vi "SLAM_Testing.vi"() -> ()   [LabVIEW 2012]
uses:
  <vilib>/DAQmx/write.llb/DAQmx Write.vi
  <vilib>/DAQmx/write.llb/DAQmx Write (Digital 1D Bool NChan 1Samp 1Line).vi
  <vilib>/DAQmx/configure/task.llb/DAQmx Clear Task.vi
  <vilib>/DAQmx/create/task.llb/DAQmx Create Task.vi
  <vilib>/DAQmx/configure/task.llb/DAQmx Start Task.vi
  <vilib>/DAQmx/create/channels.llb/DAQmx Create Virtual Channel.vi
  <vilib>/DAQmx/create/channels.llb/DAQmx Create Channel (DO-Digital Output).vi
  <vilib>/DAQmx/miscellaneous.llb/DAQmx Fill In Error Info.vi
panel:
  in  "File Name":string
  in  "Save Enable":bool
  in  "Timed Relay Control":bool
  in  "ECOLAB Button":bool
  in  "Tab Control":enum32{"MAIN", "  CONFIG  "}(tab)
  out "Flow2 Wayne":dbl
  out "Vol Percent":dbl format="%.1f"
  in  "Save When Running?":bool=TRUE
  out "Ave FLOW Ratio":dbl format="%.1f"
  out "Ave VDC2":dbl format="%.1f"
  out "Ave VDC1":dbl format="%.1f"
  out "VOLTAGE 2":dbl format="%.1f"
  out "FLOW 2":u32
  in  "ENABLE OUTPUT":bool
  in  "Time Setpoint [s]":dbl=10.0
  in  "START/RESET":bool
  out "MASS 1":dbl format="%.1f"
  out "MASS 2":dbl format="%.1f"
  out "VOLTAGE 1":dbl format="%.1f"
  out "Elapsed Time [s]":dbl format="%.1f"
  out "Output":bool
  out "FLOW 1":u32
  in  "Reset Flow 1":bool
  in  "Reset Flow 2":bool
  in  "Average Interval [sec]":dbl=0.1
  in  "X Seconds":dbl=3.0
  out "Ave Size":i32=86
  out "Flow1 Wayne":dbl
  in  "DAQ TAB":T1(tab)=enum."9237"
  in  "Save Interval [s]":dbl=1.0 min=0.0
  in  "Folder Location":path
  out "Save Error":errorcluster
  out "File Path":path
  in  "Scale Template":T2={"Channel Select"=0, "Clear/Reset Scales"=FALSE, "Channel #"=["0", "1", "2", "3", "4", "5"], "Scale Names"=["0", "1", "2", "3", "4", "5"], "Set?"=[FALSE, FALSE, FALSE, FALSE, FALSE, FALSE, FALSE, FALSE, FALSE, FALSE, FALSE, FALSE], "HI/LO Setpoints"=[1.0, 0.0, 1.0, 0.0, 1.0, 0.0, 1.0, 0.0, 1.0, 0.0, 1.0, 0.0], "Units"=["0", "1", "2", "3", "4", "5"], "HI/LO Signals"=[1.0, 0.0, 1.0, 0.0, 1.0, 0.0, 1.0, 0.0, 1.0, 0.0, 1.0, 0.0], "Slope/Intercept"=[1.0, 0.0, 1.0, 0.0, 1.0, 0.0, 1.0, 0.0, 1.0, 0.0, 1.0, 0.0], "IN/OUT Values"=[0.0, 0.0, 0.0, 0.0, 0.0, 0.0, 0.0, 0.0, 0.0, 0.0, 0.0, 0.0], "Sim Signals?"=FALSE, "Sim. Signal"=0.0} {"Sim. Signal" format="%#.3p"; "Channel Select" min=0 step=1; "Slope/Intercept" format="%#.3p"; "HI/LO Setpoints" format="%#.3p"; "IN/OUT Values" format="%#.3p"; "HI/LO Signals" format="%#.3p"}
  in  "9237 Name":tag="9237"
  in  "9237 Config":T3={"Sample Rate [Hz]"=25000.0, "Number of Samples"=2500, "Max Value [V]"=0.025, "Min Value [V]"=-0.025, "Voltage Excitation Source"=10200, "Ext. Excitation Value (VDC)"=10.0, "Sample Timing Index"=0, "Cut-Off [Hz]"=1.0, "HI/LO Trim [%]"=10.0, "Near Stable Threshold [V]"=1e-06, "Near Stable Change Limit [V]"=5e-07, "Stable Threshold [V]"=2.5e-08, "Stable Change Limit [V]"=1e-10, "Rolling Average"=4} {"Voltage Excitation Source" items=["Internal"=10200, "External"=10167, "None"=10230]; "Sample Timing Index" max=2; "Sample Rate [Hz]" format="%#_6p"; "Max Value [V]" format="%#_6p"; "Min Value [V]" format="%#_6p"; "Stable Change Limit [V]" format="%.2p"; "Stable Threshold [V]" format="%.2p"; "Near Stable Change Limit [V]" format="%.2p"; "Near Stable Threshold [V]" format="%.2p"; "Cut-Off [Hz]" format="%0.2f"}
  out "9237 Error":errorcluster={"status"=TRUE, "code"=-200077, "source"="Property Node DAQmx Timing (arg 1) in DAQmx 9237 4ch Load Cell (SubVI).vi->SLAM_Testing.vi <append>\n<B>Property: </B>SampTimingEngine\n<B>Requested Value: </B>0\n<B>You Can Select: </B>2\n\n<B>Task Name: </B>9237"}
  in  "9229 Name":tag="9229"
  in  "9229 Config":T4={"Sample Rate [Hz]"=25000.0, "Samples/Ch"=2500, "Max Value [V]"=60.0, "Min Value [V]"=0.0, "Rolling Average"=5, "HI/LO Trim [%]"=1.0, "Sample Timing Engine"=2} {"Sample Timing Engine" max=2; "Sample Rate [Hz]" min=0.0001 max=50000.0 format="%#_6p"; "Samples/Ch" min=1 step=1; "Max Value [V]" min=-60.0 max=60.0 format="%#_6p"; "Min Value [V]" min=-60.0 max=60.0 format="%#_6p"; "Rolling Average" min=1 step=1; "HI/LO Trim [%]" min=1.0 max=99.0}
  out "9229 Error":errorcluster={"status"=TRUE, "code"=-200220, "source"="SLAM_Testing.vi<append>\n<B>Device Specified: </B>9229\n<B>Suggested Device(s): </B>cDAQ5, 9237, 6009\n\n<B>Task Name: </B>9229"}
  in  "9411 Name":tag="9411"
  out "9411 Error":errorcluster={"status"=TRUE, "code"=-201003, "source"="DAQmx Create Channel (CI-Count Edges).vi:2<append>\n<B>Device Specified: </B>9411\n\n<B>Task Name: </B>9411_0"}
  in  "K-Factor Array [pulses / liter]":dbl[](array[numeric])=[1800.0, 1800.0, 1800.0, 1800.0]
  in  "Reset Array":bool[](array[boolean])=[FALSE, FALSE, FALSE, FALSE]
  out "Flow0":T5 {"Volume [gal]" format="%#.3f"; "Rate [GPM]" format="%#.3f"; "Elapsed Time [s]" format="%.1f"}
  out "Flow1":T5 {"Volume [gal]" format="%#.3f"; "Rate [GPM]" format="%#.3f"; "Elapsed Time [s]" format="%.1f"}
  out "Flow2":T5 {"Volume [gal]" format="%#.3f"; "Rate [GPM]" format="%#.3f"; "Elapsed Time [s]" format="%.1f"}
  in  "9411 Config":T6={"Digital Filter Enable"=TRUE, "Minimum Pulse Width [seconds]"=2.5e-08} {"Minimum Pulse Width [seconds]" min=2.5e-08 max=6.4e-06 format="%.3p"}
  out "Flow3":T5 {"Volume [gal]" format="%#.3f"; "Rate [GPM]" format="%#.3f"; "Elapsed Time [s]" format="%.1f"}
  in  "Relay Control (Manual)":bool[](array[boolean])=[FALSE, FALSE, FALSE, FALSE]
  out "9481 Error":errorcluster
  in  "9481 Name":tag="9481"
  in  "Stop Program":bool=TRUE
  # "Hand Care Concentrates"
  # "Save Enable"
  # "File / Test Name"
  # "Blake Otting 6-26-2013"
  # "TEST CONTROL"
  # "TEST MEASUREMENTS"
  # "LIVE MEASUREMENTS"
  # "grams"
  # "Average Values"
  # "grams"
  # "Voltage 1"
  # "vdc"
  # "Voltage 2"
  # "vdc"
  # "vdc"
  # "Volume Ratio"
  # "vdc"
  # "Flow1 / Flow2"
  # "Volume %"
  # "Flow2 / (F1+F2)"
  # "mL"
  # "Scaled Output Value"
  # "mL"
  # "Stop Saving\nN seconds after OFF"
  # "Save When Enabled\nand Running + N?"
  # "Scaled Output Value"
  # "0 = Use Manual Save Signal Only"
  # "Ch.\n#"
  # "Scale\nName"
  # "Set\nValues?"
  # "Channel\nSelect"
  # "Scaled"
  # "Pre-Scaled"
  # "Scaling Result"
  # "Values"
  # "Units"
  # "Values"
  # "HI"
  # "Slope"
  # "IN"
  # "LO"
  # "Intercept"
  # "OUT"
  # "HI"
  # "Slope"
  # "IN"
  # "LO"
  # "Intercept"
  # "OUT"
  # "HI"
  # "Slope"
  # "IN"
  # "LO"
  # "Intercept"
  # "OUT"
  # "HI"
  # "Slope"
  # "IN"
  # "LO"
  # "Intercept"
  # "OUT"
  # "DATA SAMPLE CONFIG"
  # "FILTER / SMOOTHING CONFIG"
  # "9229 Configuration"
  # "CTR0:  SRC(1)  GATE(2)  COM(12)"
  # "CTR1:  SRC(6)  GATE(7)  COM(12)"
  # "CTR2:  SRC(3)  GATE(1)  COM(12)"
  # "CTR3:  SRC(8)  GATE(6)  COM(12)"
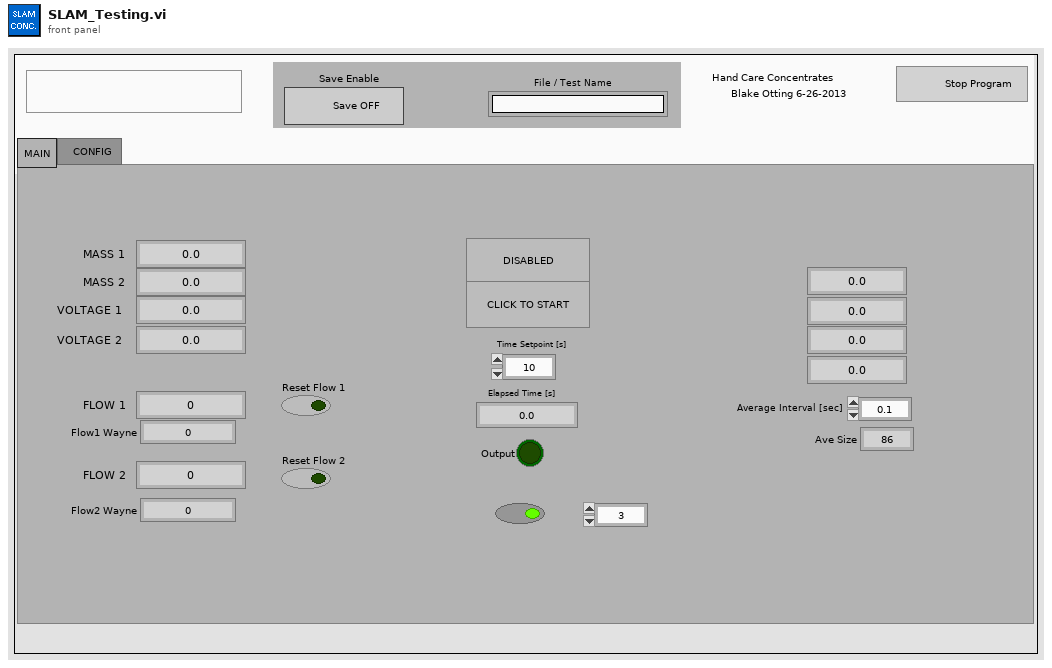
[diagram p1: front panel]
types:
  T1 = enum32{"SAVE", "SCALE", "9237", "9229", "9411", "9481"}
  T2 = cluster{"Channel Select":i32, "Clear/Reset Scales":bool, "Channel #":string[], "Scale Names":string[], "Set?":bool[], "HI/LO Setpoints":dbl[], "Units":string[], "HI/LO Signals":dbl[], "Slope/Intercept":dbl[], "IN/OUT Values":dbl[], "Sim Signals?":bool, "Sim. Signal":dbl}
  T3 = cluster{"Sample Rate [Hz]":dbl, "Number of Samples":i32, "Max Value [V]":dbl, "Min Value [V]":dbl, "Voltage Excitation Source":i32, "Ext. Excitation Value (VDC)":dbl, "Sample Timing Index":u32, "Cut-Off [Hz]":dbl, "HI/LO Trim [%]":dbl, "Near Stable Threshold [V]":dbl, "Near Stable Change Limit [V]":dbl, "Stable Threshold [V]":dbl, "Stable Change Limit [V]":dbl, "Rolling Average":i32}
  T4 = cluster{"Sample Rate [Hz]":dbl, "Samples/Ch":i32, "Max Value [V]":dbl, "Min Value [V]":dbl, "Rolling Average":i32, "HI/LO Trim [%]":dbl, "Sample Timing Engine":u32}
  T5 = cluster{"Pulse Count":u32, "Volume [mL]":u32, "Volume [gal]":dbl, "Rate [GPM]":dbl, "Elapsed Time [s]":dbl}
  T6 = cluster{"Digital Filter Enable":bool, "Minimum Pulse Width [seconds]":dbl}
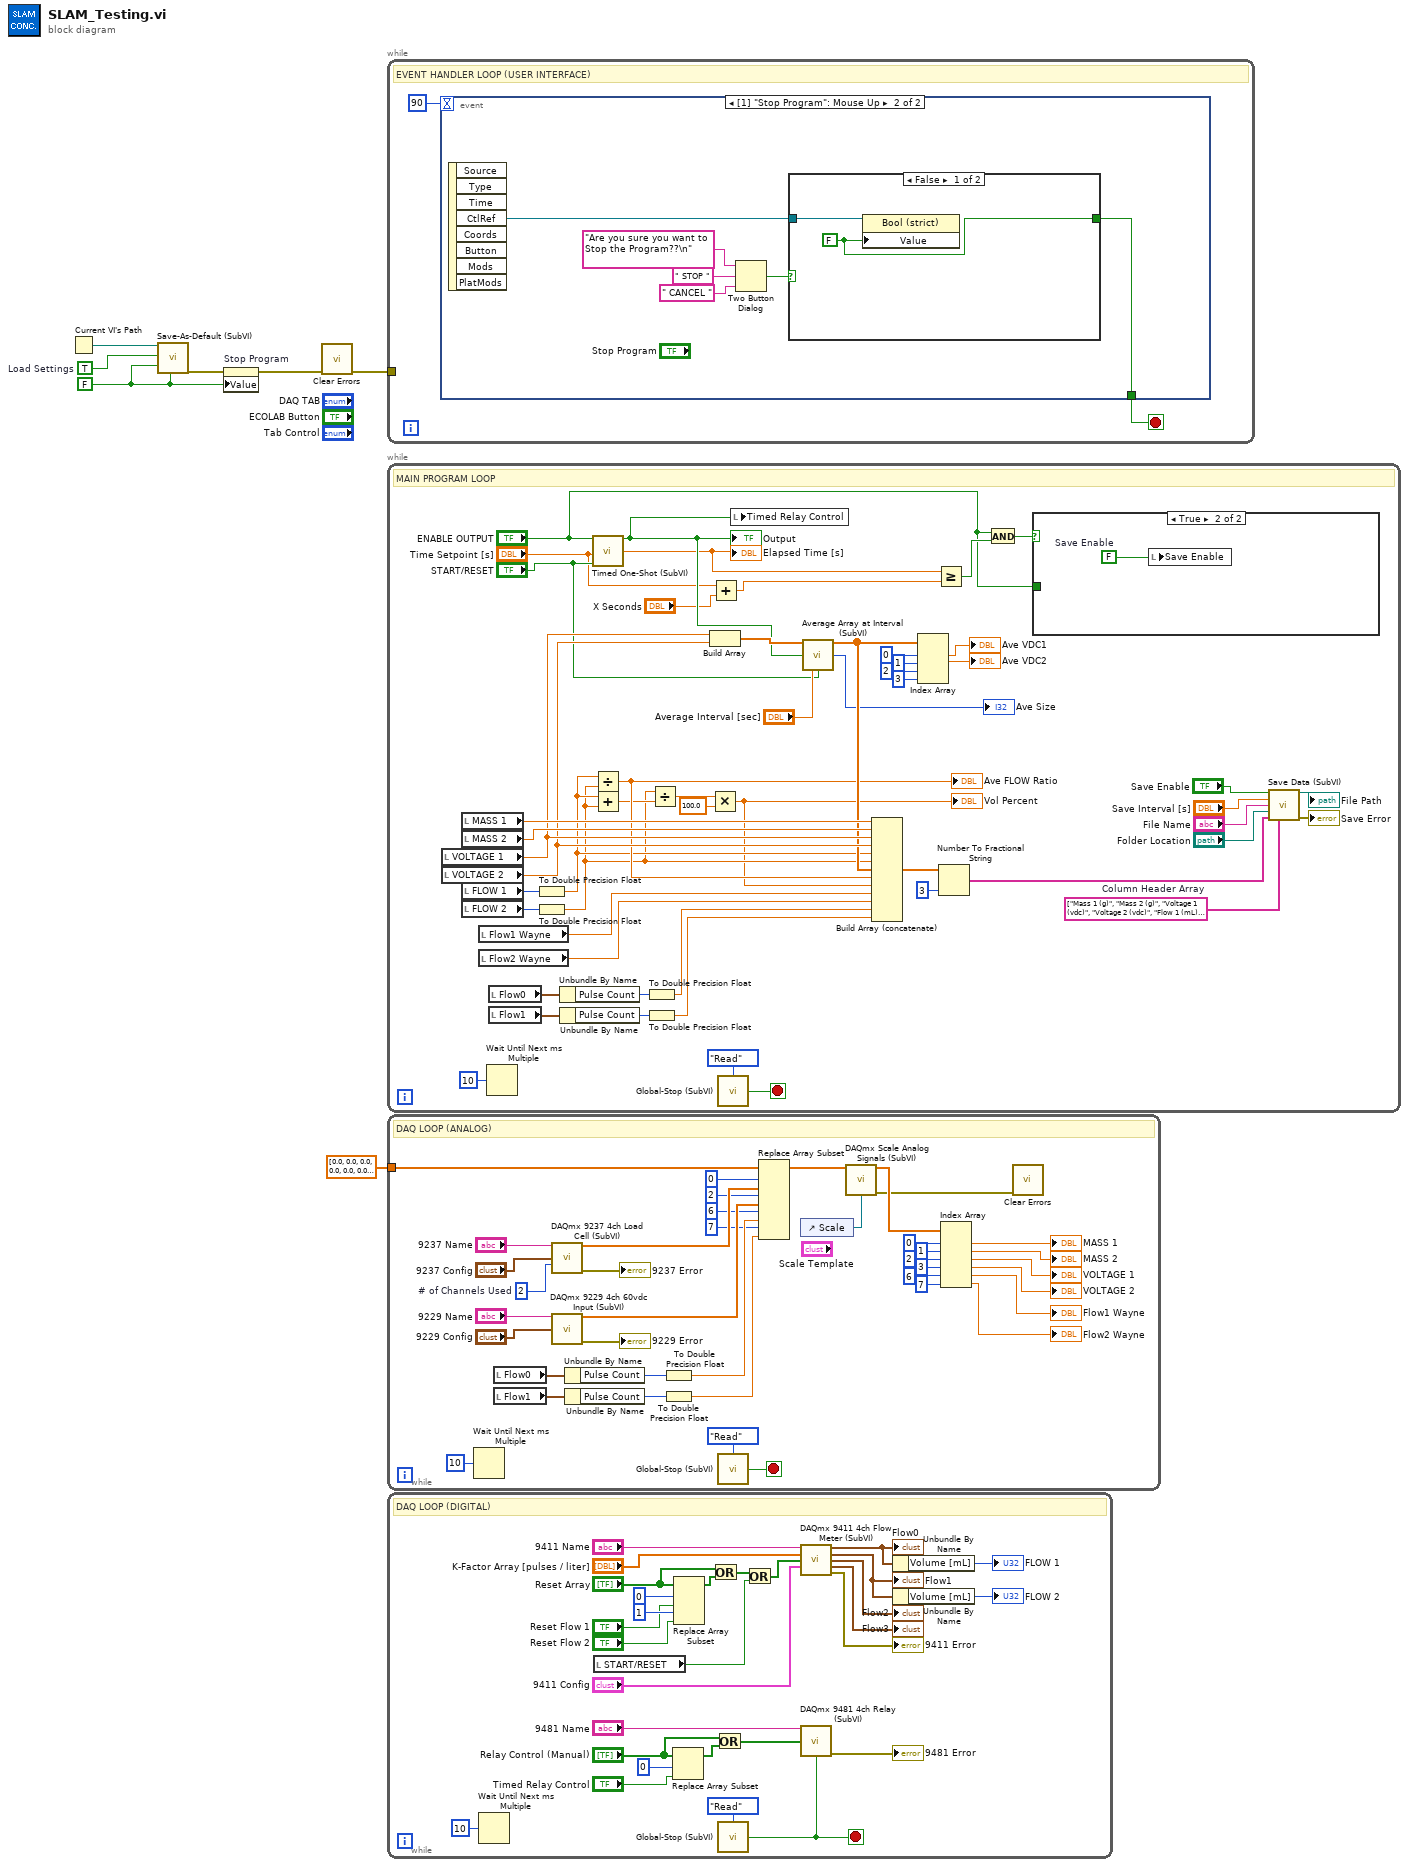
[diagram p0: block diagram]
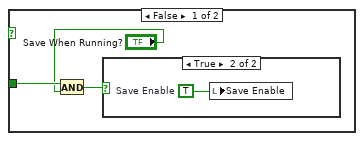
[diagram p2: hidden frame]
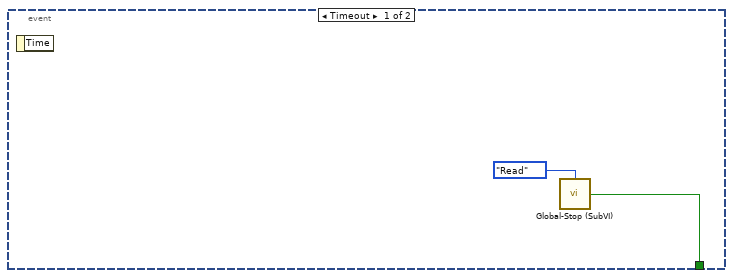
[diagram p4: hidden frame]
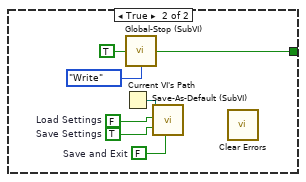
[diagram p5: hidden frame]
diagram:
  w4 = TRUE  # Load Settings
  w2 = FALSE
  n1 = Current VI's Path() -> (path=w5:path)
  n2 = call "Save-As-Default (SubVI).vi"("Current VI's Path"=w5, "Load Settings"=w4, "Save Settings"=w2, "Save and Exit"=w2) -> ("Save as Default Error"=w3:errorcluster)  [unwired: 15 in]
  n3 = property on="Stop Program" class="Bool (strict)"(error in=w3, "Value"=w2) -> (error out=w7:errorcluster)  [unwired: 1 in, 1 out]
  n4 = call <vilib>:"Clear Errors.vi"("error in (no error)"=w7) -> ("error out"=w6:errorcluster)  [unwired: 6 out]
  n5 = while {
    tunnel: w6 -> [_]
    stop <- w9 stop-if-true
    # "EVENT HANDLER LOOP (USER INTERFACE)"
    n6 = event shown="[1] \"Stop Program\": Mouse Up" {
      selector: _ -> [_ _]
      dyn-events: _ -> [_ _]
      timeout: 90 -> [_ _]
      tunnel: [w10 w13] -> w9
      event Timeout {
        n7 = event-data() -> ()  [unwired: 2 out]
        n8 = call "Global-Stop (SubVI).vi"("Mode (Read)"=enum16{"Read", "Write"}."Read") -> ("OUT"=w10:bool)  [unwired: 3 in]
      }
      event "Stop Program": Mouse Up {
        n9 = event-data() -> ("CtlRef"=w12:refnum<vi>)  [unwired: 8 out]
        n10 = Two Button Dialog(message="Are you sure you want to Stop the Program??\n", 1:" CANCEL " ("F button name (\"Cancel\")"), 2:" STOP ") -> (T button?=w14:bool)
        n11 = case shown="False" w14 {
          tunnel: [w18 w24] -> w13
          tunnel: w12 -> [w19 _]
          frame False {
            w18 = FALSE ("Value")
            n12 = property class="Bool (strict)"(reference=w19, "Value"=w18) -> ()  [unwired: 1 in, 2 out]
          }
          frame True {
            w20 = FALSE  # Save and Exit
            w21 = TRUE  # Save Settings
            w22 = FALSE  # Load Settings
            n13 = Current VI's Path() -> (path=w23:path)
            n14 = call "Global-Stop (SubVI).vi"("Mode (Read)"=enum16{"Read", "Write"}."Write", "IN"=TRUE) -> ("OUT"=w24:bool)  [unwired: 2 in]
            n15 = call "Save-As-Default (SubVI).vi"("Current VI's Path"=w23, "Load Settings"=w22, "Save Settings"=w21, "Save and Exit"=w20) -> ()  [unwired: 15 in, 1 out]
            n16 = call <vilib>:"Clear Errors.vi"() -> ()  [unwired: 1 in, 7 out]
          }
        }
      }
    }
  }
  n17 = while {
    stop <- w78 stop-if-true
    w68 = string[] ["Mass 1 (g)", "Mass 2 (g)", "Voltage 1 (vdc)", "Voltage 2 (vdc)", "Flow 1 (mL)", "Flow 2 (mL)", "Ave VDC1", "Ave VDC2", "Ave Flow Ratio", "Ave Percentage", "Flow1 Wayne", "Flow2 Wayne", "Flow0 Raw Pulse", "Flow1 Raw Pulse"]  # Column Header Array
    # "MAIN PROGRAM LOOP"
    n18 = local read "VOLTAGE 1"() -> (w62:dbl)
    n19 = local read "VOLTAGE 2"() -> (w61:dbl)
    n20 = local read "MASS 1"() -> (w76:dbl)
    n21 = local read "MASS 2"() -> (w75:dbl)
    n22 = local read "FLOW 1"() -> (w74:u32)
    n23 = local read "FLOW 2"() -> (w73:u32)
    n24 = local read "Flow1 Wayne"() -> (w32:dbl)
    n25 = local read "Flow2 Wayne"() -> (w31:dbl)
    n26 = Wait Until Next ms Multiple(millisecond multiple=u32 10) -> ()  [unwired: 1 out]
    n27 = local read "Flow0"() -> (w33:T5)
    n28 = local read "Flow1"() -> (w34:T5)
    n29 = To Double Precision Float(number=w74) -> (double precision float=w40:dbl)
    n30 = To Double Precision Float(number=w73) -> (double precision float=w38:dbl)
    n31 = Unbundle By Name(w33) -> ("Pulse Count"=w30:u32)
    n32 = Unbundle By Name(w34) -> ("Pulse Count"=w29:u32)
    n33 = call "Timed One-Shot (SubVI).vi"("ENABLE OUTPUT"="ENABLE OUTPUT", "Time Setpoint [s]"="Time Setpoint [s]", "START/RESET"="START/RESET") -> ("Output"=w50:bool, "Elapsed Time [s]"=w49:dbl)  [unwired: 11 in]
    "Elapsed Time [s]" <- w49
    "Output" <- w50
    n34 = Divide(x=w40, y=w38) -> (x/y=w41:dbl)
    "Ave FLOW Ratio" <- w41
    n35 = Add(x=w40, y=w38) -> (x+y=w39:dbl)
    n36 = To Double Precision Float(number=w30) -> (double precision float=w28:dbl)
    n37 = To Double Precision Float(number=w29) -> (double precision float=w27:dbl)
    n38 = Divide(x=w38, y=w39) -> (x/y=w37:dbl)
    n39 = Build Array(w62, w61) -> (w60:dbl[])
    n40 = Multiply(x=w37, y=100.0) -> (x*y=w35:dbl)
    "Vol Percent" <- w35
    n41 = Add(x="Time Setpoint [s]", y="X Seconds") -> (x+y=w45:dbl)
    n42 = call "Global-Stop (SubVI).vi"("Mode (Read)"=enum16{"Read", "Write"}."Read") -> ("OUT"=w78:bool)  [unwired: 3 in]
    n43 = local write "Timed Relay Control"(w50) -> ()
    n44 = call "Average Array at Interval (SubVI).vi"("Signals IN"=w60, "Enable"=w50, "Sample Interval [sec]"="Average Interval [sec]", "Reset Averages"="START/RESET") -> ("Signals OUT"=w53:dbl[], "Ave Size"=→"Ave Size":i32)  [unwired: 10 in]
    n45 = Build Array (concatenate)(w76, w75, w62, w61, w40, w38, w53, w41, w35, w32, w31, w28, w27) -> (w64:dbl[])
    n46 = Index Array(array=w53, index #1=0, index #2=1, index #3=2, index #4=3) -> (element #1=→"Ave VDC1":dbl, element #2=→"Ave VDC2":dbl)  [unwired: 2 out]
    n47 = Greater Or Equal?(x=w49, y=w45) -> (x >= y?=w44:bool)
    n48 = Number To Fractional String(number=w64, precision (6)=i16 3) -> (F-format string=w70:string[])  [unwired: 2 in]
    n49 = And(x="ENABLE OUTPUT", y=w44) -> (x .and. y?=w43:bool)
    n50 = case shown="True" w43 {
      tunnel: "ENABLE OUTPUT" -> [w82 _]
      frame False {
        n51 = And(x=w82, y="Save When Running?") -> (x .and. y?=w80:bool)
        n52 = case shown="True" w80 {
          frame False {
          }
          frame True {
            w83 = TRUE  # Save Enable
            n53 = local write "Save Enable"(w83) -> ()
          }
        }
      }
      frame True {
        w84 = FALSE  # Save Enable
        n54 = local write "Save Enable"(w84) -> ()
      }
    }
    n55 = call "Save Data (SubVI).vi"("Save Enable"="Save Enable", "Save Interval [sec]"="Save Interval [s]", "File Name"="File Name", "Folder Location"="Folder Location", "Data Array (Row)"=w70, "Column Header Array"=w68) -> ("File Path"=→"File Path":path, "Save Error"=→"Save Error":errorcluster)  [unwired: 7 in, 1 out]
  }
  n56 = while {
    tunnel: dbl[] [0.0, 0.0, 0.0, 0.0, 0.0, 0.0, 0.0, 0.0] -> [w113]
    stop <- w122 stop-if-true
    w99 = 2  # # of Channels Used
    # "DAQ LOOP (ANALOG)"
    n57 = Wait Until Next ms Multiple(millisecond multiple=u32 10) -> ()  [unwired: 1 out]
    n58 = local read "Flow0"() -> (w86:T5)
    n59 = local read "Flow1"() -> (w85:T5)
    n60 = call "DAQmx 9237 4ch Load Cell (SubVI).vi"("9237 Name"="9237 Name", "9237 Config"="9237 Config", "# of Channels Used"=w99) -> ("Filtered Signals"=w121:dbl[], "9237 Error"=→"9237 Error":errorcluster)  [unwired: 8 in, 3 out]
    n61 = call "DAQmx 9229 4ch 60vdc Input (SubVI).vi"("9229 Name"="9229 Name", "9229 Config"="9229 Config") -> ("Measurements"=w117:dbl[], "9229 Error"=→"9229 Error":errorcluster)  [unwired: 12 in]
    n62 = Unbundle By Name(w86) -> ("Pulse Count"=w95:u32)
    n63 = Unbundle By Name(w85) -> ("Pulse Count"=w93:u32)
    n64 = To Double Precision Float(number=w95) -> (double precision float=w94:dbl)
    n65 = To Double Precision Float(number=w93) -> (double precision float=w91:dbl)
    n66 = call "Global-Stop (SubVI).vi"("Mode (Read)"=enum16{"Read", "Write"}."Read") -> ("OUT"=w122:bool)  [unwired: 3 in]
    n67 = Replace Array Subset(array=w113, new element #1=w121, index #1=0, new element #2=w117, index #2=2, new element #3=w94, index #3=6, new element #4=w91, index #4=7) -> (w111:dbl[])
    n68 = control-ref of="Scale"() -> (w112:refnum<vi>)
    n69 = call "DAQmx Scale Analog Signals (SubVI).vi"("Measured Signals"=w111, "Scale Reference"=w112) -> ("Scaled Values"=w110:dbl[], "Scale Error"=w100:errorcluster)  [unwired: 12 in]
    n70 = Index Array(array=w110, index #1=0, index #2=1, index #3=2, index #4=3, index #5=6, index #6=7) -> (element #1=→"MASS 1":dbl, element #2=→"MASS 2":dbl, element #3=→"VOLTAGE 1":dbl, element #4=→"VOLTAGE 2":dbl, element #5=→"Flow1 Wayne":dbl, element #6=→"Flow2 Wayne":dbl)
    n71 = call <vilib>:"Clear Errors.vi"("error in (no error)"=w100) -> ()  [unwired: 6 in, 1 out]
  }
  n72 = while {
    stop <- w150 stop-if-true
    # "DAQ LOOP (DIGITAL)"
    n73 = Wait Until Next ms Multiple(millisecond multiple=u32 10) -> ()  [unwired: 1 out]
    n74 = local read "START/RESET"() -> (w125:bool)
    n75 = Replace Array Subset(array="Relay Control (Manual)", new element="Timed Relay Control", index=0) -> (w130:bool[])
    n76 = Replace Array Subset(array="Reset Array", new element #1="Reset Flow 1", index #1=0, new element #2="Reset Flow 2", index #2=1) -> (w136:bool[])
    n77 = Or(x="Reset Array", y=w136) -> (x .or. y?=w126:bool[])
    n78 = Or(x="Relay Control (Manual)", y=w130) -> (x .or. y?=w132:bool[])
    n79 = call "Global-Stop (SubVI).vi"("Mode (Read)"=enum16{"Read", "Write"}."Read") -> ("OUT"=w150:bool)  [unwired: 3 in]
    n80 = Or(x=w126, y=w125) -> (x .or. y?=w124:bool[])
    n81 = call "DAQmx 9411 4ch Flow Meter (SubVI).vi"("9411 Name"="9411 Name", "K-Factor Array [pulses / liter]"="K-Factor Array [pulses / liter]", "Reset Array"=w124, "9411 Config"="9411 Config") -> ("Flow0"=w141:T5, "Flow1"=w142:T5, "Flow2"=→"Flow2":T5, "Flow3"=→"Flow3":T5, "9411 Error"=→"9411 Error":errorcluster)  [unwired: 7 in]
    "Flow0" <- w141
    "Flow1" <- w142
    n82 = call "DAQmx 9481 4ch Relay (SubVI).vi"("9481 Name"="9481 Name", "Relay Control"=w132, "Stop Program"=w150) -> ("9481 Error"=→"9481 Error":errorcluster)  [unwired: 12 in]
    n83 = Unbundle By Name(w141) -> ("Volume [mL]"=→"FLOW 1":u32)
    n84 = Unbundle By Name(w142) -> ("Volume [mL]"=→"FLOW 2":u32)
  }
